vi "IRDriver.vi"(7 "Port":T1 {"Port" items=["Port 1", "Port 2", "Port 3", "Port 4"]; "MUX Port" items=["No MUX", "MUX 1", "MUX 2", "MUX 3", "MUX 4"]}, 11 "NXT In":T3) -> (2 "Sector (0-9)":i16, 3 "NXT Out":T3 caption="NXT")   [LabVIEW 2012]
uses:
  <vilib>/NXT/Subs/LVHSConnector.ctl
  <vilib>/NXT/LegoClasses/BrickReference/BrickReference.lvclass
  <vilib>/NXT/HiTechnic/HiTechnic Controls/HiTechnic Port.ctl
  <vilib>/NXT/Block Support/NXT_InputPort.ctl
  <vilib>/NXT/HiTechnic/HiTechnic SubVIs/HiTechnic IRSeeker Sensor_AC dir.vi
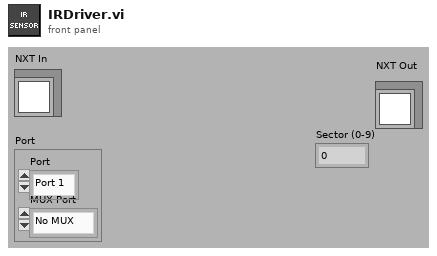
[diagram p1: front panel]
types:
  T1 = typedef "HiTechnic Port.ctl" = cluster{"Port":T2, "MUX Port":u8}
  T2 = typedef "NXT_InputPort.ctl" = u8
  T3 = typedef "LVHSConnector.ctl" = refnum<class "BrickReference.lvclass">
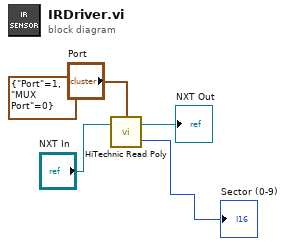
[diagram p0: block diagram]
diagram:
  (unwired) T1 {"Port"=1, "MUX Port"=0} ("Port/MUX")
  n1 = call-poly <vilib>:"HiTechnic Read Poly.vi"("NXT"="NXT In", "Port/MUX"="Port") -> ("Direction (0-9)"=→"Sector (0-9)":i16, "NXT"=→"NXT Out":T3)  [unwired: 1 in]
